vi "Teleop.vi"(1 "PreValue 2":bool, 3 "PreValue":bool, 9 "PreValue 3":bool, 10 "Match Info":T1={"Autonomous Elapsed Seconds"=0.0, "TeleOp Elapsed Seconds"=0.0, "Disabled Elapsed Seconds"=0.0, "Visited Autonomous"=FALSE, "Visited TeleOp"=FALSE, "Visited Disabled"=FALSE, "Autonomous Settings"={"Autonomous Style"=enum."Independent", "VI Refnum"=refnum}}, 11 "Call Context":T2) -> (0 "CurrentValue 2":bool, 2 "CurrentValue":bool, 8 "CurrentValue 3":bool)   [LabVIEW 2015]
doc: "This VI is called for each TeleOp packet received from the DS where the robot is not disabled. It is often used to read from the joysticks and update I/O or to update setpoints for timed control loops. It should complete and return within 20 milliseconds or it may miss DS packets."
uses:
  <vilib>/Rock Robotics/WPI/DriverStation/WPI_DriverStationDerivedRobotMode.ctl
  <vilib>/Rock Robotics/WPI/DriverStation/WPI_DriverStationMatch Info.ctl
  <vilib>/Rock Robotics/WPI/Solenoid/WPI_SolenoidValue.ctl
  <vilib>/Rock Robotics/WPI/Utilities/WPI_GetSetVariantRefNum.vi
  <vilib>/Rock Robotics/Network Tables/NT Write Boolean.vi
  <vilib>/Rock Robotics/Network Tables/NT Write Numeric Array.vi
  <vilib>/Rock Robotics/Network Tables/NT Read Boolean.vi
  <vilib>/Rock Robotics/Network Tables/NT Read Number.vi
  <vilib>/Rock Robotics/WPI/Solenoid/WPI_SolenoidSetEnum.vi
panel:
  out "Sample Slider 0":dbl(slide) scale=0.0..5.0
  out "Sample Boolean 1":bool
  out "Sample Boolean 0":bool
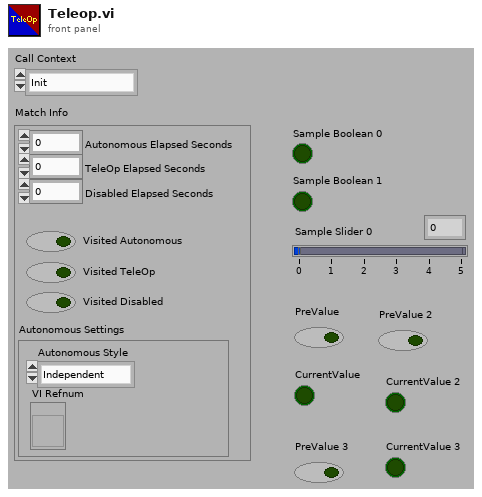
[diagram p1: front panel]
types:
  T1 = typedef "WPI_DriverStationMatch Info.ctl" = cluster{"Autonomous Elapsed Seconds":dbl, "TeleOp Elapsed Seconds":dbl, "Disabled Elapsed Seconds":dbl, "Visited Autonomous":bool, "Visited TeleOp":bool, "Visited Disabled":bool, "Autonomous Settings":cluster{"Autonomous Style":enum16{"Iterative", "Independent"}, "VI Refnum":refnum<vi>}}
  T2 = typedef "WPI_DriverStationDerivedRobotMode.ctl" = enum16{"Init", "Execute", "Stop"}
  T3 = typedef "WPI_SolenoidValue.ctl" = enum16{"Off", "On", "Forward", "Reverse"}
  T4 = typedef "WPI_JoystickDevRef.ctl" = cluster{"Device":T5}
  T5 = typedef "WPI_JoystickDeviceEnum.ctl" = enum16{"USB 0", "USB 1", "USB 2", "USB 3", "USB 4", "USB 5"}
  T6 = cluster{"Buttons[0]":bool, "Buttons[1]":bool, "Buttons[2]":bool, "Buttons[3]":bool, "Buttons[4]":bool, "Buttons[5]":bool, "Buttons[6]":bool, "Buttons[7]":bool, "Buttons[8]":bool}
  T7 = typedef "WPI_ServoDeviceRef.ctl" = cluster{"DeviceStatus":errorcluster, "PWM Channel":T8, "DeadBand":T9}
  T8 = typedef "FPGA_DIOPWMChannel.ctl" = enum8{"PWM 0", "PWM 1", "PWM 2", "PWM 3", "PWM 4", "PWM 5", "PWM 6", "PWM 7", "PWM 8", "PWM 9", "PWM MXP 0", "PWM MXP 1", "PWM MXP 2", "PWM MXP 3", "PWM MXP 4", "PWM MXP 5", "PWM MXP 6", "PWM MXP 7", "PWM MXP 8", "PWM MXP 9", "Invalid"}
  T9 = typedef "WPI_PWMDeadband.ctl" = cluster{"Name":string, "maxPositivePwm":i32, "minPositivePwm":i32, "centerPwm":i32, "maxNegativePwm":i32, "minNegativePwm":i32, "angularRange":u16}
  T10 = typedef "WPI_RobotDriveDevRef.ctl" = cluster{"DevStatus":errorcluster, "Motors[]":T11[], "Square Inputs":bool, "Max Output":dbl}
  T11 = typedef "WPI_MotorControlDeviceRef.ctl" = cluster{"DeviceStatus":errorcluster, "Type":T12, "PWM":cluster{"PWM Channel":T8, "DeadBand":T9}, "CAN":cluster{"Device Number":u8, "Control Mode":T13, "Semaphore":T14, "Max Vout":dbl, "TalonSRX Control Mode":T15}, "Invert":bool}
  T12 = typedef "WPI_MotorControlType.ctl" = enum16{"PWM", "CAN", "CANTalonSRX"}
  T13 = typedef "WPI_CANJaguar_ControlMode.ctl" = enum8{"Percent VBus", "Current", "Speed", "Position", "Voltage"}
  T14 = typedef "Semaphore RefNum" = refnum<k1>
  T15 = typedef "WPI_CANTalonSRX_APIControlMode.ctl" = enum8{"Percent VBus", "Speed", "Position", "Slave", "Unchanged / Invalid", "Voltage Compensation", "Current", "Motion Profile"}
  T16 = typedef "WPI_SolenoidDevRef.ctl" = cluster{"DevStatus":errorcluster, "Pneumatics Control Module":u8, "Forward Solenoid Channel":T17, "Reverse Solenoid Channel":T17}
  T17 = typedef "WPI_SolenoidChannel.ctl" = enum8{"Solenoid 0", "Solenoid 1", "Solenoid 2", "Solenoid 3", "Solenoid 4", "Solenoid 5", "Solenoid 6", "Solenoid 7", "Invalid"}
  T18 = typedef "WPI_DigitalInputDevRef.ctl" = cluster{"DevStatus":errorcluster, "DIO Channel":T19}
  T19 = typedef "FPGA_DIOChannel.ctl" = enum8{"DIO 0", "DIO 1", "DIO 2", "DIO 3", "DIO 4", "DIO 5", "DIO 6", "DIO 7", "DIO 8", "DIO 9", "DIO MXP 0", "DIO MXP 1", "DIO MXP 2", "DIO MXP 3", "DIO MXP 4", "DIO MXP 5", "DIO MXP 6", "DIO MXP 7", "DIO MXP 8", "DIO MXP 9", "DIO MXP 10", "DIO MXP 11", "DIO MXP 12", "DIO MXP 13", "DIO MXP 14", "DIO MXP 15", "Invalid"}
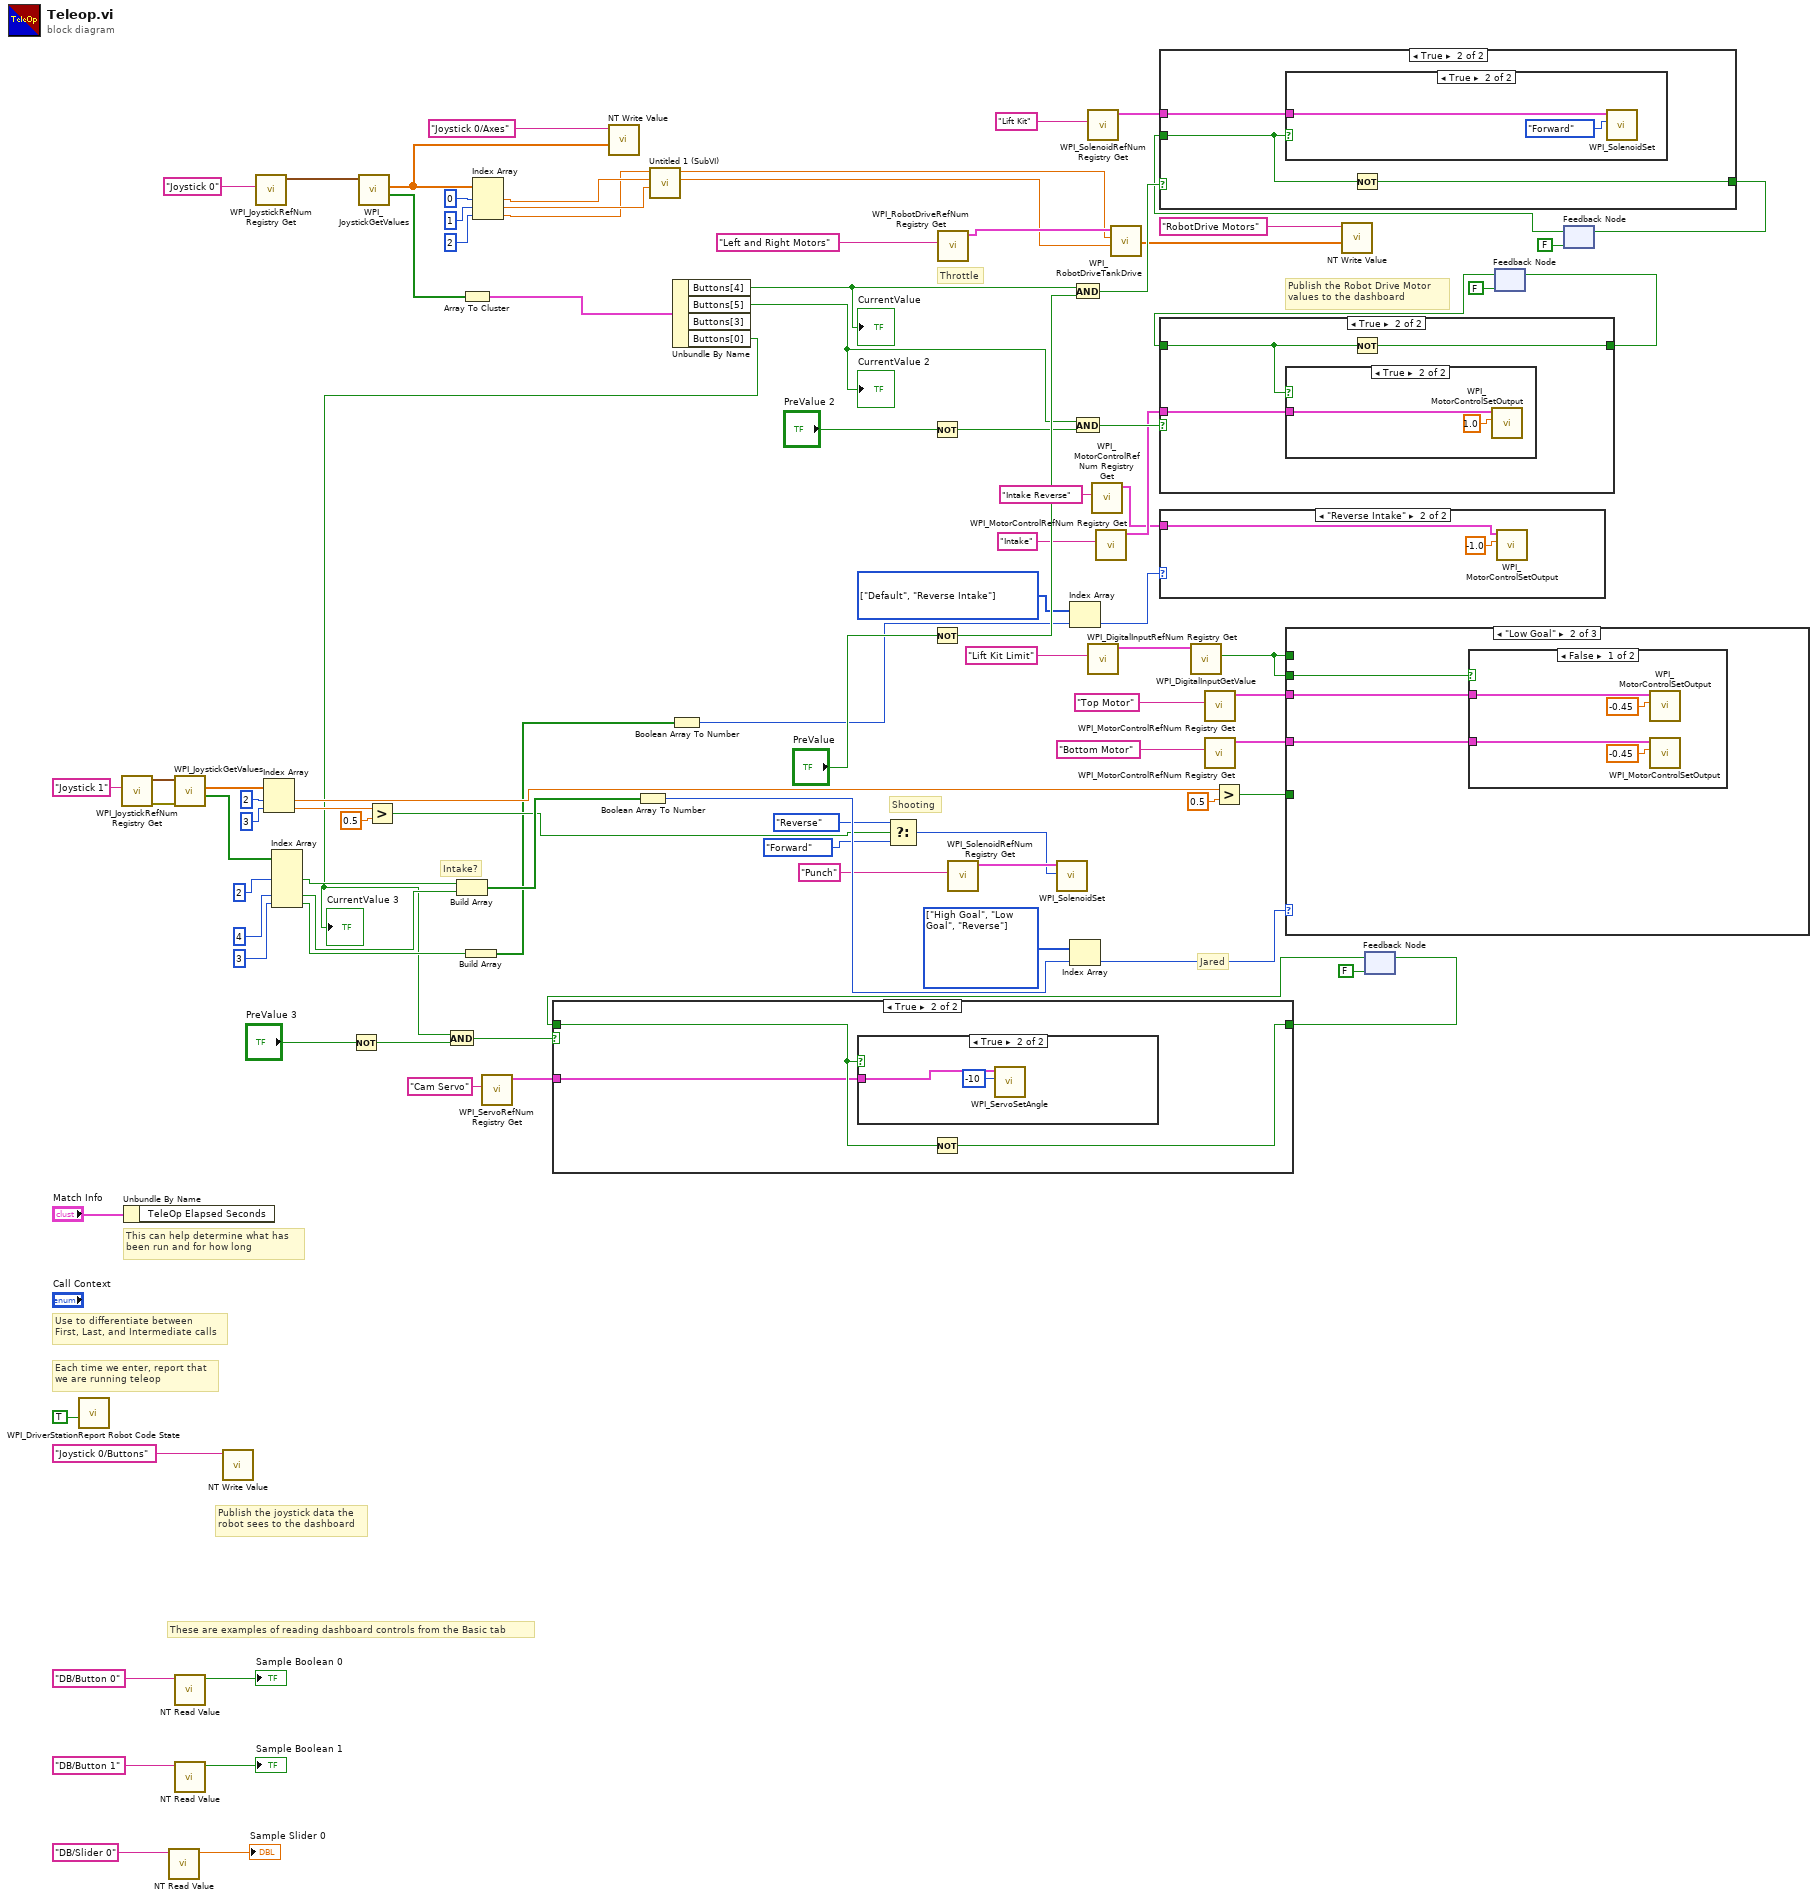
[diagram p0: block diagram]
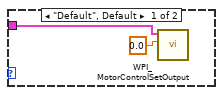
[diagram p2: hidden frame]
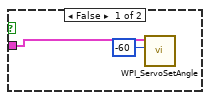
[diagram p4: hidden frame]
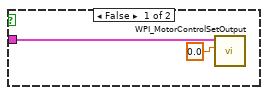
[diagram p6: hidden frame]
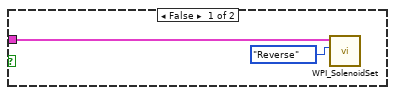
[diagram p8: hidden frame]
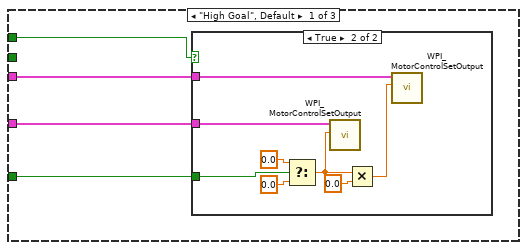
[diagram p9: hidden frame]
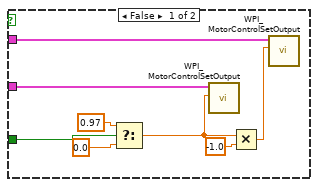
[diagram p10: hidden frame]
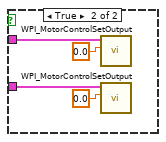
[diagram p11: hidden frame]
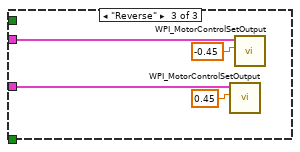
[diagram p12: hidden frame]
diagram:
  w15 = enum16{"Default", "Reverse Intake"}[] [enum."Default", enum."Reverse Intake"] items=["Default", "Reverse Intake"] ("array")
  w77 = enum16{"High Goal", "Low Goal", "Reverse", ""}[] [enum."High Goal", enum."Low Goal", enum."Reverse"] items=["High Goal", "Low Goal", "Reverse", ""] ("array")
  # "Jared"
  # "Intake?"
  # "Shooting"
  # "Throttle"
  # "These are examples of reading dashboard controls from the Basic tab"
  # "Publish the Robot Drive Motor\nvalues to the dashboard"
  # "Publish the joystick data the\nrobot sees to the dashboard"
  # "Each time we enter, report that\nwe are running teleop"
  # "Use to differentiate between\nFirst, Last, and Intermediate calls"
  # "This can help determine what has\nbeen run and for how long"
  n1 = call <vilib>:"WPI_DriverStationReport Robot Code State.vi"("TeleOp"=TRUE ("Autonomous")) -> ()  [unwired: 10 in, 1 out]
  n2 = call <vilib>:"WPI_JoystickRefNum Registry Get.vi"("refnum name"="Joystick 1") -> ("error out"=w58:errorcluster, "JoystickDevRef"=w57:T4)  [unwired: 1 in, 8 out]
  n3 = Unbundle By Name("Match Info") -> ()  [unwired: 1 out]
  n4 = call-poly <vilib>:"NT Read Value.vi"("Name"="DB/Slider 0" ("refnum name")) -> ("Numeric"=→"Sample Slider 0":dbl)  [unwired: 9 in, 1 out]
  n5 = call <vilib>:"WPI_JoystickGetValues.vi"("error in (no error)"=w58, "JoystickDevRef"=w57) -> ("Buttons"=w26:bool[], "Axes"=w55:dbl[])  [unwired: 5 in, 3 out]
  n6 = call-poly <vilib>:"NT Read Value.vi"("Name"="DB/Button 0" ("refnum name")) -> ("Boolean"=→"Sample Boolean 0":bool)  [unwired: 9 in, 1 out]
  n7 = call-poly <vilib>:"NT Read Value.vi"("Name"="DB/Button 1" ("refnum name")) -> ("Boolean"=→"Sample Boolean 1":bool)  [unwired: 9 in, 1 out]
  n8 = call-poly <vilib>:"NT Write Value.vi"("Name"="Joystick 0/Buttons") -> ()  [unwired: 10 in, 1 out]
  n9 = call <vilib>:"WPI_JoystickRefNum Registry Get.vi"("refnum name"="Joystick 0") -> ("JoystickDevRef"=w92:T4)  [unwired: 1 in, 9 out]
  n10 = Index Array(array=w55, index #1=2 ("index"), index #2=3 ("index")) -> (element #1=w54:dbl, element #2=w49:dbl)
  n11 = Index Array(array=w26, index #2=2 ("index"), index #4=4 ("index"), index #5=3 ("index")) -> (element #2=w32:bool, element #4=w30:bool, element #5=w17:bool)  [unwired: 2 in, 2 out]
  n12 = Not(x="PreValue 3") -> (.not. x?=w38:bool)
  n13 = call <vilib>:"WPI_JoystickGetValues.vi"("JoystickDevRef"=w92) -> ("Buttons"=w73:bool[], "Axes"=w88:dbl[])  [unwired: 6 in, 3 out]
  n14 = Greater?(x=w49, y=0.5) -> (0:w21:bool)
  n15 = Build Array(w32, w30) -> (w79:bool[])
  n16 = Array To Cluster(array=w73) -> (cluster=w80:T6)
  n17 = Build Array(w17) -> (w16:bool[])
  n18 = Index Array(array=w88, index #1=0 ("index"), index #2=1 ("index"), index #3=2 ("index")) -> (element #1=w10:dbl, element #2=w11:dbl, element #3=w9:dbl)
  n19 = call <vilib>:"WPI_ServoRefNum Registry Get.vi"("refnum name"="Cam Servo") -> ("ServoDeviceRef"=w5:T7)  [unwired: 9 in, 1 out]
  n20 = call-poly <vilib>:"NT Write Value.vi"("Numeric Array"=w88, "Name"="Joystick 0/Axes") -> ()  [unwired: 9 in, 1 out]
  n21 = Boolean Array To Number(Boolean array=w79) -> (number=w78:u32)
  n22 = call "Untitled 1 (SubVI).vi"("upper limit 2"=w11, "upper limit"=w10, "Throttle"=w9) -> ("Numeric 2"=w1:dbl, "Numeric"=w2:dbl)  [unwired: 7 in]
  n23 = Boolean Array To Number(Boolean array=w16) -> (number=w19:u32)
  n24 = Unbundle By Name(w80) -> ("Buttons[4]"=w70:bool, "Buttons[5]"=w43:bool, "Buttons[0]"=w3:bool)  [unwired: 1 out]
  "CurrentValue" <- w70
  "CurrentValue 2" <- w43
  "CurrentValue 3" <- w3
  n25 = And(x=w3, y=w38) -> (x .and. y?=w37:bool)
  n26 = Select(t=WPI_SolenoidValue."Reverse" ("Value"), s=w21, f=WPI_SolenoidValue."Forward" ("Value")) -> (s? t:f=w24:T3)
  n27 = Not(x="PreValue 2") -> (.not. x?=w42:bool)
  n28 = Not(x="PreValue") -> (.not. x?=w68:bool)
  n29 = call <vilib>:"WPI_RobotDriveRefNum Registry Get.vi"("refnum name"="Left and Right Motors") -> ("RobotDriveDevRef"=w7:T10)  [unwired: 1 in, 9 out]
  n30 = call <vilib>:"WPI_SolenoidRefNum Registry Get.vi"("refnum name"="Punch") -> ("SolenoidDevRef"=w25:T16)  [unwired: 9 in, 1 out]
  n31 = call-poly <vilib>:"WPI_SolenoidSet.vi"("Value"=w24, "SolenoidDevRef"=w25) -> ()  [unwired: 8 in, 2 out]
  n32 = Index Array(array=w15, index=w19) -> (element=w14:enum16{"Default", "Reverse Intake"})
  n33 = Index Array(array=w77, index=w78) -> (element=w76:enum16{"High Goal", "Low Goal", "Reverse", ""})
  n34 = And(x=w70, y=w68) -> (x .and. y?=w67:bool)
  n35 = And(x=w43, y=w42) -> (x .and. y?=w41:bool)
  n36 = call <vilib>:"WPI_SolenoidRefNum Registry Get.vi"("refnum name"="Lift Kit") -> ("SolenoidDevRef"=w62:T16)  [unwired: 9 in, 1 out]
  n37 = call <vilib>:"WPI_DigitalInputRefNum Registry Get.vi"("refnum name"="Lift Kit Limit") -> ("DigitalInputDevRef"=w29:T18)  [unwired: 9 in, 1 out]
  n38 = call <vilib>:"WPI_MotorControlRefNum Registry Get.vi"("refnum name"="Intake Reverse") -> ("MotorControlDevRef"=w13:T11)  [unwired: 9 in, 1 out]
  n39 = call <vilib>:"WPI_MotorControlRefNum Registry Get.vi"("refnum name"="Intake") -> ("MotorControlDevRef"=w20:T11)  [unwired: 9 in, 1 out]
  n40 = call <vilib>:"WPI_RobotDriveTankDrive.vi"("Right axis value"=w1, "Left axis value"=w2, "RobotDriveDevRef"=w7) -> ("Motor Values"=w8:dbl[])  [unwired: 6 in, 2 out]
  n41 = case shown="\"Reverse Intake\"" w14 {
    tunnel: w13 -> [w96 w98]
    frame "Default", Default {
      n42 = call <vilib>:"WPI_MotorControlSetOutput.vi"("Output"=0.0, "MotorControlDevRef"=w96) -> ()  [unwired: 7 in, 3 out]
    }
    frame "Reverse Intake" {
      n43 = call <vilib>:"WPI_MotorControlSetOutput.vi"("Output"=-1.0, "MotorControlDevRef"=w98) -> ()  [unwired: 7 in, 3 out]
    }
  }
  n44 = call <vilib>:"WPI_DigitalInputGetValue.vi"("DigitalInputDevRef"=w29) -> ("Value"=w27:bool)  [unwired: 8 in, 2 out]
  n45 = call <vilib>:"WPI_MotorControlRefNum Registry Get.vi"("refnum name"="Top Motor") -> ("MotorControlDevRef"=w71:T11)  [unwired: 9 in, 1 out]
  n46 = call <vilib>:"WPI_MotorControlRefNum Registry Get.vi"("refnum name"="Bottom Motor") -> ("MotorControlDevRef"=w75:T11)  [unwired: 9 in, 1 out]
  n47 = Greater?(x=w54, y=0.5) -> (0:w52:bool)
  n48 = case shown="\"Low Goal\"" w76 {
    tunnel: w75 -> [w103 w122 w133]
    tunnel: w71 -> [w102 w121 w131]
    tunnel: w52 -> [w101 _ _]
    tunnel: w27 -> [_ w120 _]
    tunnel: w27 -> [w100 _ _]
    frame "High Goal", Default {
      n49 = case shown="True" w100 {
        tunnel: w103 -> [w105 w119]
        tunnel: w102 -> [w104 w118]
        tunnel: w101 -> [w110 w117]
        frame False {
          n50 = Select(t=0.97, s=w110, f=0.0) -> (s? t:f=w109:dbl)
          n51 = call <vilib>:"WPI_MotorControlSetOutput.vi"("Output"=w109, "MotorControlDevRef"=w105) -> ()  [unwired: 7 in, 3 out]
          n52 = Multiply(x=w109, y=-1.0) -> (x*y=w111:dbl)
          n53 = call <vilib>:"WPI_MotorControlSetOutput.vi"("Output"=w111, "MotorControlDevRef"=w104) -> ()  [unwired: 7 in, 3 out]
        }
        frame True {
          n54 = Select(t=0.0, s=w117, f=0.0) -> (s? t:f=w115:dbl)
          n55 = call <vilib>:"WPI_MotorControlSetOutput.vi"("Output"=w115, "MotorControlDevRef"=w119) -> ()  [unwired: 7 in, 3 out]
          n56 = Multiply(x=w115, y=0.0) -> (x*y=w113:dbl)
          n57 = call <vilib>:"WPI_MotorControlSetOutput.vi"("Output"=w113, "MotorControlDevRef"=w118) -> ()  [unwired: 7 in, 3 out]
        }
      }
    }
    frame "Low Goal" {
      n58 = case shown="False" w120 {
        tunnel: w122 -> [w123 w129]
        tunnel: w121 -> [w124 w127]
        frame False {
          n59 = call <vilib>:"WPI_MotorControlSetOutput.vi"("Output"=-0.45, "MotorControlDevRef"=w124) -> ()  [unwired: 7 in, 3 out]
          n60 = call <vilib>:"WPI_MotorControlSetOutput.vi"("Output"=-0.45, "MotorControlDevRef"=w123) -> ()  [unwired: 7 in, 3 out]
        }
        frame True {
          n61 = call <vilib>:"WPI_MotorControlSetOutput.vi"("Output"=0.0, "MotorControlDevRef"=w127) -> ()  [unwired: 7 in, 3 out]
          n62 = call <vilib>:"WPI_MotorControlSetOutput.vi"("Output"=0.0, "MotorControlDevRef"=w129) -> ()  [unwired: 7 in, 3 out]
        }
      }
    }
    frame "Reverse" {
      n63 = call <vilib>:"WPI_MotorControlSetOutput.vi"("Output"=0.45, "MotorControlDevRef"=w133) -> ()  [unwired: 7 in, 3 out]
      n64 = call <vilib>:"WPI_MotorControlSetOutput.vi"("Output"=-0.45, "MotorControlDevRef"=w131) -> ()  [unwired: 7 in, 3 out]
    }
  }
  n65 = call-poly <vilib>:"NT Write Value.vi"("Numeric Array"=w8, "Name"="RobotDrive Motors") -> ()  [unwired: 9 in, 1 out]
  n66 = feedback #1(FALSE) -> (w34:bool)
  n67 = case shown="True" w37 {
    tunnel: [w135 w138] -> w35
    tunnel: w34 -> [w135 w137]
    tunnel: w5 -> [_ w136]
    frame False {
    }
    frame True {
      n68 = case shown="True" w137 {
        tunnel: w136 -> [w140 w142]
        frame False {
          n69 = call <vilib>:"WPI_ServoSetAngle.vi"("Angle"=-60, "ServoDeviceRef"=w140) -> ()  [unwired: 8 in, 2 out]
        }
        frame True {
          n70 = call <vilib>:"WPI_ServoSetAngle.vi"("Angle"=-10, "ServoDeviceRef"=w142) -> ()  [unwired: 8 in, 2 out]
        }
      }
      n71 = Not(x=w137) -> (.not. x?=w138:bool)
    }
  }
  n72 = feedback-in #1(w35) -> ()
  n73 = feedback #2(FALSE) -> (w45:bool)
  n74 = case shown="True" w41 {
    tunnel: [w143 w146] -> w46
    tunnel: w45 -> [w143 w144]
    tunnel: w20 -> [_ w145]
    frame False {
    }
    frame True {
      n75 = case shown="True" w144 {
        tunnel: w145 -> [w148 w150]
        frame False {
          n76 = call <vilib>:"WPI_MotorControlSetOutput.vi"("Output"=0.0, "MotorControlDevRef"=w148) -> ()  [unwired: 7 in, 3 out]
        }
        frame True {
          n77 = call <vilib>:"WPI_MotorControlSetOutput.vi"("Output"=1.0, "MotorControlDevRef"=w150) -> ()  [unwired: 7 in, 3 out]
        }
      }
      n78 = Not(x=w144) -> (.not. x?=w146:bool)
    }
  }
  n79 = feedback-in #2(w46) -> ()
  n80 = feedback #3(FALSE) -> (w64:bool)
  n81 = case shown="True" w67 {
    tunnel: [w151 w154] -> w65
    tunnel: w64 -> [w151 w152]
    tunnel: w62 -> [_ w153]
    frame False {
    }
    frame True {
      n82 = case shown="True" w152 {
        tunnel: w153 -> [w156 w158]
        frame False {
          n83 = call-poly <vilib>:"WPI_SolenoidSet.vi"("Value"=WPI_SolenoidValue."Reverse", "SolenoidDevRef"=w156) -> ()  [unwired: 8 in, 2 out]
        }
        frame True {
          n84 = call-poly <vilib>:"WPI_SolenoidSet.vi"("Value"=WPI_SolenoidValue."Forward", "SolenoidDevRef"=w158) -> ()  [unwired: 8 in, 2 out]
        }
      }
      n85 = Not(x=w152) -> (.not. x?=w154:bool)
    }
  }
  n86 = feedback-in #3(w65) -> ()
